vi "picoquant_get_count_rates.vi"(8 "error in (no error)":errorcluster, 11 "picoquant_generic in":refnum<class "picoquant_generic.lvclass">) -> (0 "error out":errorcluster, 2 "count_rates":T1, 3 "picoquant_generic out":refnum<class "picoquant_generic.lvclass">)   [LabVIEW 2015, in "picoquant_generic.lvclass"]
uses:
  picoquant_generic.lvclass
  Hydraharp/hydraharp/hydraharp_count_rates.ctl
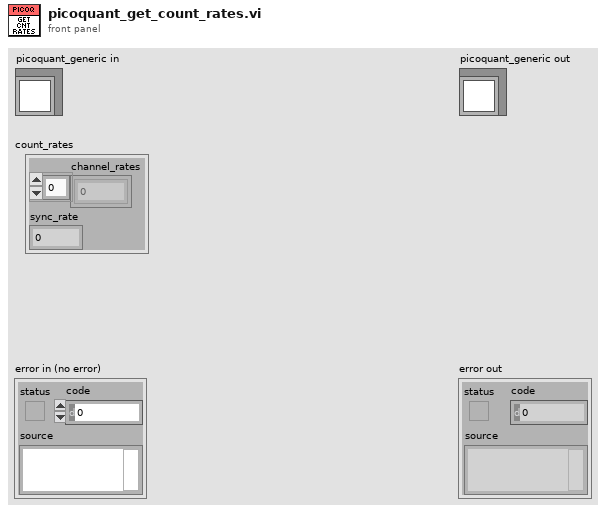
[diagram p1: front panel]
types:
  T1 = typedef "hydraharp_count_rates.ctl" = cluster{"channel_rates":i32[], "sync_rate":i32}
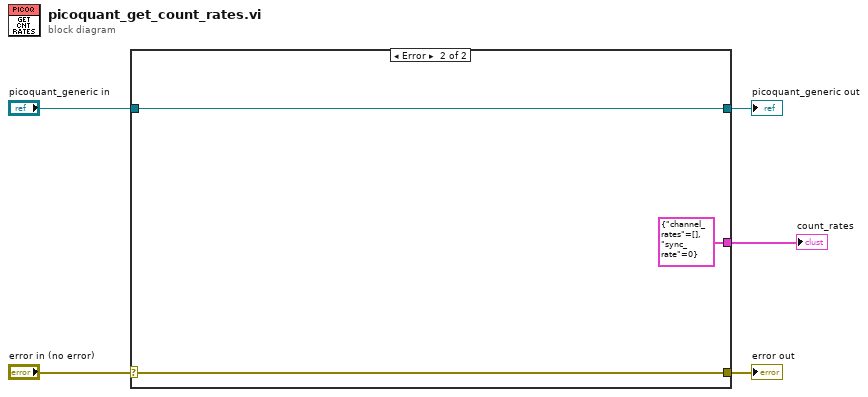
[diagram p0: block diagram]
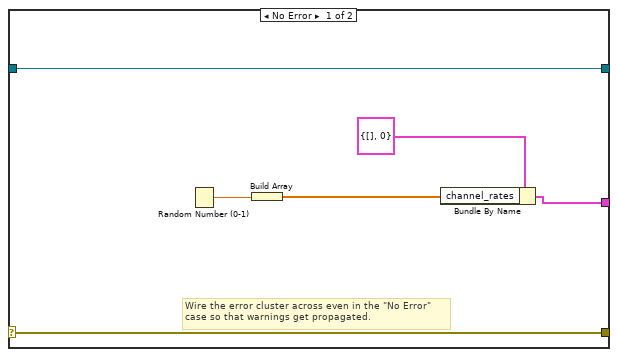
[diagram p2: hidden frame]
diagram:
  n1 = case shown="Error" "error in (no error)" {
    selector: "error in (no error)" -> [w10 w14]
    tunnel: [w10 w14] -> w4
    tunnel: [w11 w13] -> w2
    tunnel: "picoquant_generic in" -> [w11 w13]
    tunnel: [w6 T1 {"channel_rates"=[], "sync_rate"=0} ("count_rates")] -> w1
    frame No Error {
      # "Wire the error cluster across even in the \"No Error\"\ncase so that warnings get propagated."
      n2 = Random Number (0-1)() -> (number: 0 to 1=w8:dbl)
      n3 = Build Array(w8) -> (w7:dbl[])
      n4 = Bundle By Name(cluster=T1 {"channel_rates"=[], "sync_rate"=0} ("count_rates"), "channel_rates"=w7) -> (w6:T1)
    }
    frame Error {
    }
  }
  "error out" <- w4
  "picoquant_generic out" <- w2
  "count_rates" <- w1
